vi "TSCAN_Search.vi"(10 "字符串":string, 11 "数组":string[][](array[string])) -> (3 "数值":i32)   [LabVIEW 2019]
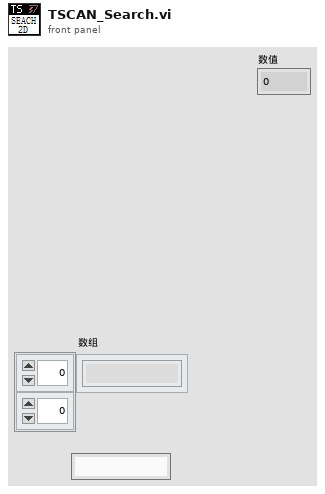
[diagram p1: front panel]
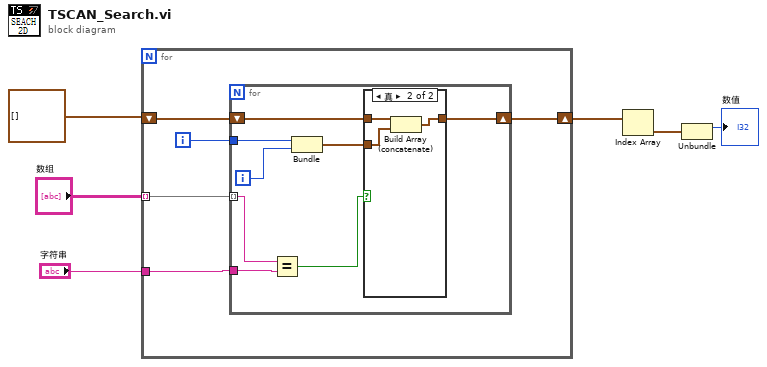
[diagram p0: block diagram]
diagram:
  n1 = for {
    tunnel: "数组" -> [w9] mode=indexing
    shift-right: [w10] -> w3
    shift-left: cluster{i32, i32}[] [] -> [w11]
    tunnel: "字符串" -> [w8]
    i -> [w7]
    n2 = for {
      shift-right: [w19] -> w10
      shift-left: w11 -> [w18]
      tunnel: w9 -> [w17] mode=indexing
      tunnel: w8 -> [w16]
      tunnel: w7 -> [w14]
      i -> [w13]
      n3 = Equal?(x=w17, y=w16) -> (x = y?=w15:bool)
      n4 = Bundle(w14, w13) -> (w12:cluster{i32, i32})  [unwired: 1 in]
      n5 = case shown="真" w15 {
        tunnel: [w20 w21] -> w19
        tunnel: w18 -> [w20 w23]
        tunnel: w12 -> [_ w22]
        frame False {
        }
        frame True {
          n6 = Build Array (concatenate)(w23, w22) -> (w21:cluster{i32, i32}[])
        }
      }
    }
  }
  n7 = Index Array(array=w3) -> (element=w2:cluster{i32, i32})  [unwired: 1 in]
  n8 = Unbundle(w2) -> (→"数值":i32)  [unwired: 1 out]
